vi "4155C Config I Stress.vi"(0 "VISA session":refnum<visa-resource-name>, 1 "IDG":dbl min=0.0 max=100000000000.0 format="%.15e", 2 "VDG compliance":dbl min=0.0 max=100000000000.0 format="%.15e", 3 "error in (no error)":errorcluster, 4 "Display on/off":bool) -> (5 "dup VISA resource name":refnum<visa-resource-name>, 6 "error out":errorcluster)   [LabVIEW 2016]
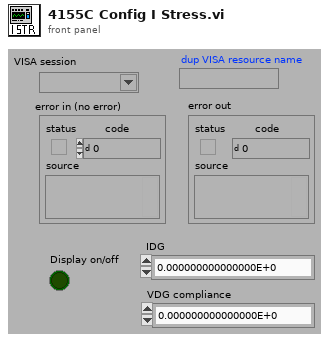
[diagram p1: front panel]
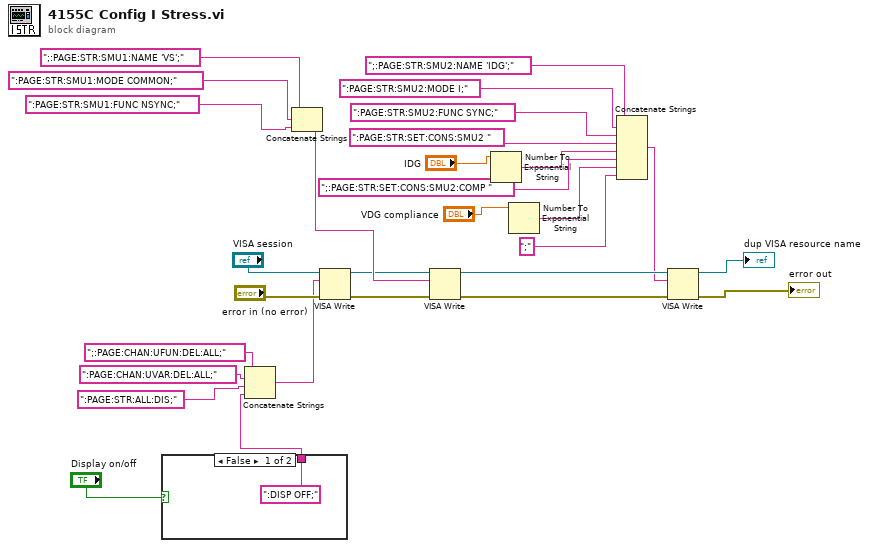
[diagram p0: block diagram]
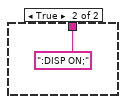
[diagram p2: hidden frame]
diagram:
  n1 = case shown="False" "Display on/off" {
    tunnel: [":DISP OFF;" ("write buffer (\"\")") ":DISP ON;" ("write buffer (\"\")")] -> w23
    frame False {
    }
    frame True {
    }
  }
  n2 = Concatenate Strings(";:PAGE:CHAN:UFUN:DEL:ALL;", ":PAGE:CHAN:UVAR:DEL:ALL;", ":PAGE:STR:ALL:DIS;", w23) -> (w24:string)
  n3 = Concatenate Strings(";:PAGE:STR:SMU1:NAME 'VS';", ":PAGE:STR:SMU1:MODE COMMON;", ":PAGE:STR:SMU1:FUNC NSYNC;") -> (w8:string)
  n4 = VISA Write(VISA resource name="VISA session", write buffer=w24, error in (no error)="error in (no error)") -> (VISA resource name out=w7:refnum<visa-resource-name>, error out=w6:errorcluster)  [unwired: 1 out]
  n5 = VISA Write(VISA resource name=w7, write buffer=w8, error in (no error)=w6) -> (VISA resource name out=w29:refnum<visa-resource-name>, error out=w28:errorcluster)  [unwired: 1 out]
  n6 = Number To Exponential String(number="IDG") -> (E-format string=w13:string)  [unwired: 3 in]
  n7 = Number To Exponential String(number="VDG compliance") -> (E-format string=w11:string)  [unwired: 3 in]
  n8 = Concatenate Strings(";:PAGE:STR:SMU2:NAME 'IDG';", ":PAGE:STR:SMU2:MODE I;", ":PAGE:STR:SMU2:FUNC SYNC;", ":PAGE:STR:SET:CONS:SMU2 ", w13, ";:PAGE:STR:SET:CONS:SMU2:COMP ", w11, ";" ("Substring")) -> (w5:string)
  n9 = VISA Write(VISA resource name=w29, write buffer=w5, error in (no error)=w28) -> (VISA resource name out=→"dup VISA resource name":refnum<visa-resource-name>, error out=→"error out":errorcluster)  [unwired: 1 out]
